vi "frameBifurcate.vi"(2 "error in (no error)":errorcluster, 3 "H2F Frame":string) -> (0 "error out":errorcluster, 1 "Bifurcated Recieved Data":T1)   [LabVIEW 2018]
uses:
  TypeDefs/recDataClust.ctl
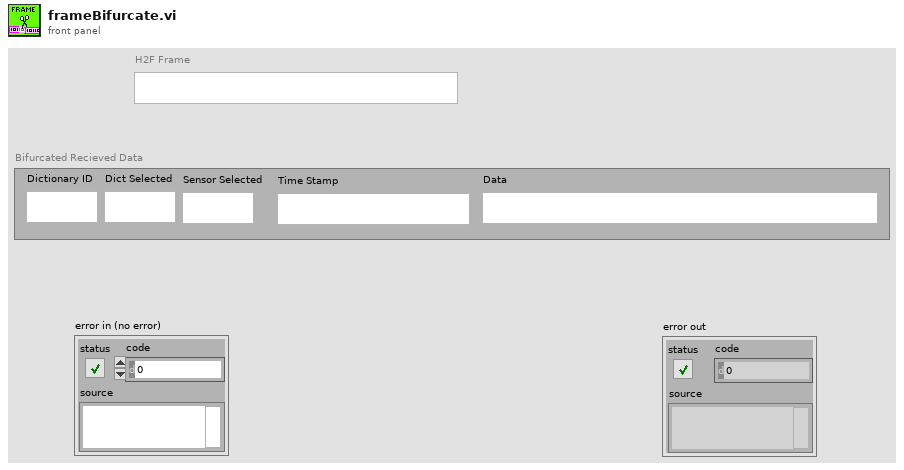
[diagram p1: front panel]
types:
  T1 = typedef "recDataClust.ctl" = cluster{"Dictionary ID":string, "Dict Selected":string, "Sensor Selected":string, "Time Stamp":string, "Data":string}
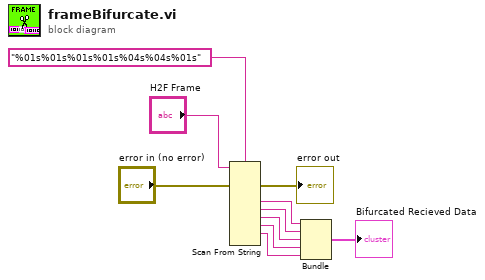
[diagram p0: block diagram]
diagram:
  n1 = Scan From String(format string="%01s%01s%01s%01s%04s%04s%01s", input string="H2F Frame", error in="error in (no error)") -> (error out=→"error out":errorcluster, output 2=w6:string, output 3=w5:string, output 4=w4:string, output 5=w3:string, output 6=w2:string)  [unwired: 10 in, 2 out]
  n2 = Bundle(w6, w5, w4, w3, w2) -> (→"Bifurcated Recieved Data":cluster{string, string, string, string, string})  [unwired: 1 in]
